vi "GetDependenciesJKI.Robot.SMO.vi"(8 "error in (no error)":errorcluster, 11 "JKI.Robot.SMO.APITesterUI in":refnum<class "JKI.Robot.SMO.APITesterUI.lvclass">) -> (0 "error out":errorcluster, 2 "JKI.Robot":refnum<class "JKI.Robot.SMO.Base.lvclass">, 3 "JKI.Robot.SMO.APITesterUI out":refnum<class "JKI.Robot.SMO.APITesterUI.lvclass">)   [LabVIEW 2015, in "JKI.Robot.SMO.APITesterUI.lvclass"]
uses:
  JKI.Robot.SMO.APITesterUI.lvclass
  JKI.Robot.SMO.Base/JKI.Robot.SMO.Base.lvclass
  JKI.Robot.SMO.APITesterUI.lvclass/JKI.Robot.SMO.APITesterUI.ctl
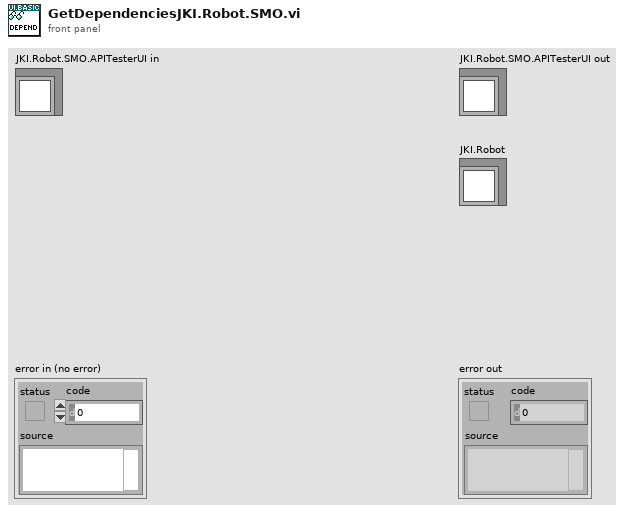
[diagram p1: front panel]
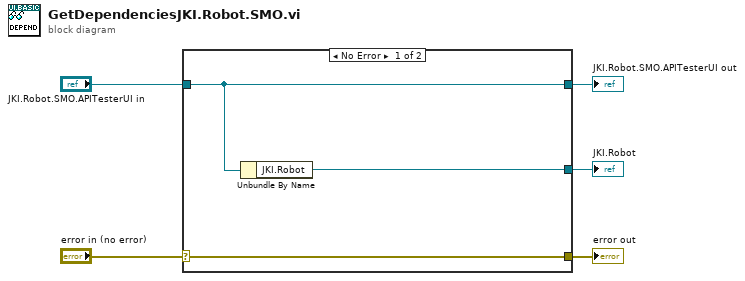
[diagram p0: block diagram]
diagram:
  n1 = case shown="No Error" "error in (no error)" {
    selector: "error in (no error)" -> [w8 w9]
    tunnel: [w8 w9] -> w4
    tunnel: [w7 w10] -> w2
    tunnel: "JKI.Robot.SMO.APITesterUI in" -> [w7 w10]
    tunnel: [w6 _] -> w1
    frame No Error {
      n2 = Unbundle By Name(w7) -> ("JKI.Robot"=w6:refnum<class "JKI.Robot.SMO.Base.lvclass">)
    }
    frame Error {
    }
  }
  "error out" <- w4
  "JKI.Robot.SMO.APITesterUI out" <- w2
  "JKI.Robot" <- w1
